vi "Read Data Buffer.vi"(0 "VISA resource name":refnum<visa-resource-name>, 1 "All Data Elements (False)":bool, 2 "Timeout (30000 milliseconds)":u32=30000, 11 "error in (no error)":errorcluster) -> (4 "VISA resource name out":refnum<visa-resource-name>, 6 "Measurement Data":dbl[](array[numeric]), 8 "Timestamp":string[](array[string]), 10 "Channel":string[](array[string]), 14 "Reading Number":string[](array[string]), 15 "error out":errorcluster)   [LabVIEW 2020, in "Keithley 27XX.lvlib"]
doc: "This VI can be used to retreive data which has already been stored in the data buffer. It does not initiate a measurement.\n\nNote:\n(1) Returning all data elements requires ASCII transfers.\n\n(2) Timestamp, Channel, and Reading Number arrays will be left empty if the All Data Elements control is set to False."
uses:
  Keithley 27XX.lvlib
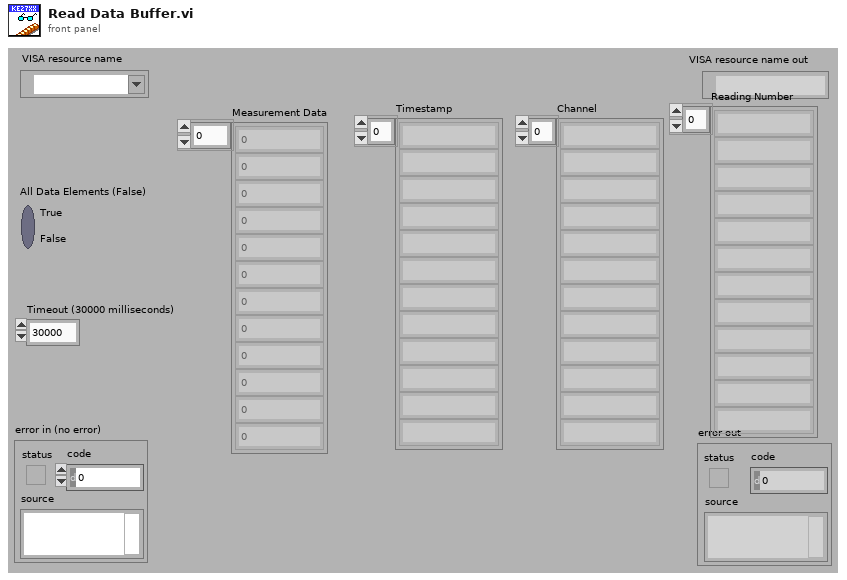
[diagram p1: front panel]
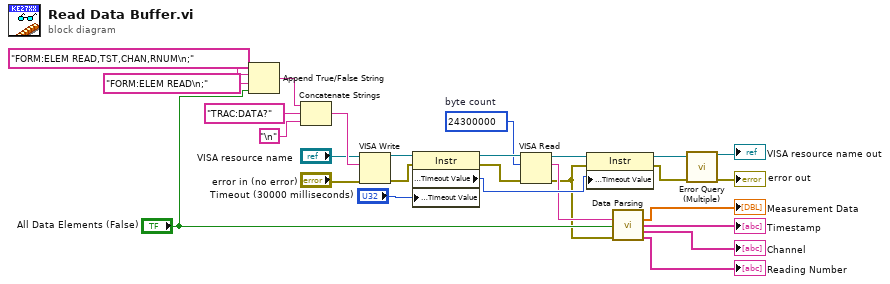
[diagram p0: block diagram]
diagram:
  w14 = u32 24300000  # byte count
  n1 = Append True/False String(1:"All Data Elements (False)", 2:"FORM:ELEM READ\n;" ("String"), 3:"FORM:ELEM READ,TST,CHAN,RNUM\n;" ("true string")) -> (0:w13:string)  [unwired: 1 in]
  n2 = Concatenate Strings(w13, "TRAC:DATA?", "\n") -> (w25:string)
  n3 = VISA Write(VISA resource name="VISA resource name", write buffer=w25, error in (no error)="error in (no error)") -> (VISA resource name out=w20:refnum<visa-resource-name>, error out=w19:errorcluster)  [unwired: 1 out]
  n4 = property class="Instr"(reference=w20, error in=w19, "General Settings:Timeout Value"="Timeout (30000 milliseconds)") -> (reference out=w18:refnum<visa-resource-name>, error out=w17:errorcluster, "General Settings:Timeout Value"=w9:u32)
  n5 = VISA Read(VISA resource name=w18, byte count=w14, error in (no error)=w17) -> (VISA resource name out=w2:refnum<visa-resource-name>, read buffer=w7:string, error out=w1:errorcluster)  [unwired: 1 out]
  n6 = property class="Instr"(reference=w2, error in=w1, "General Settings:Timeout Value"=w9) -> (reference out=w15:refnum<visa-resource-name>, error out=w16:errorcluster)
  n7 = call "Data Parsing.vi"("read buffer"=w7, "All Data Elements (False)"="All Data Elements (False)", "error in"=w1) -> ("Measurement Data"=→"Measurement Data":dbl[], "Time Stamp"=→"Timestamp":string[], "Channel"=→"Channel":string[], "Reading Number"=→"Reading Number":string[])  [unwired: 9 in]
  n8 = call "Error Query (Multiple).vi"("VISA resource name"=w15, "error in (no error)"=w16) -> ("VISA resource name out"=→"VISA resource name out":refnum<visa-resource-name>, "error out"=→"error out":errorcluster)  [unwired: 10 in, 2 out]
